vi "登陆界面.vi"(10 "引用":refnum<vi>) -> (1 "用户名":string, 2 "登陆状态":bool)   [LabVIEW 2014]
uses:
  Global.vi
panel:
  in  "退出":bool
  in  "登录":bool
  in  "密码":string
  in  "用户名":string
  # "（用户名为两位大写字母加数字组合）"
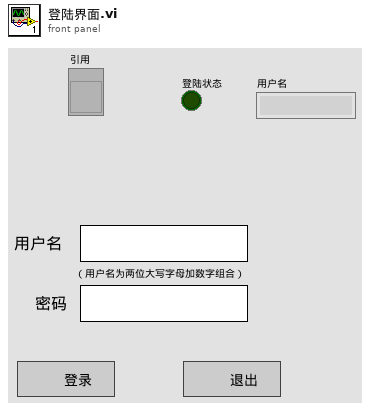
[diagram p1: front panel]
types:
  T1 = enum32{"Invalid", "Standard", "Closed", "Hidden", "Minimized", "Maximized"}
  T2 = enum8{"Enabled", "Disabled", "Disabled and Grayed Out"}
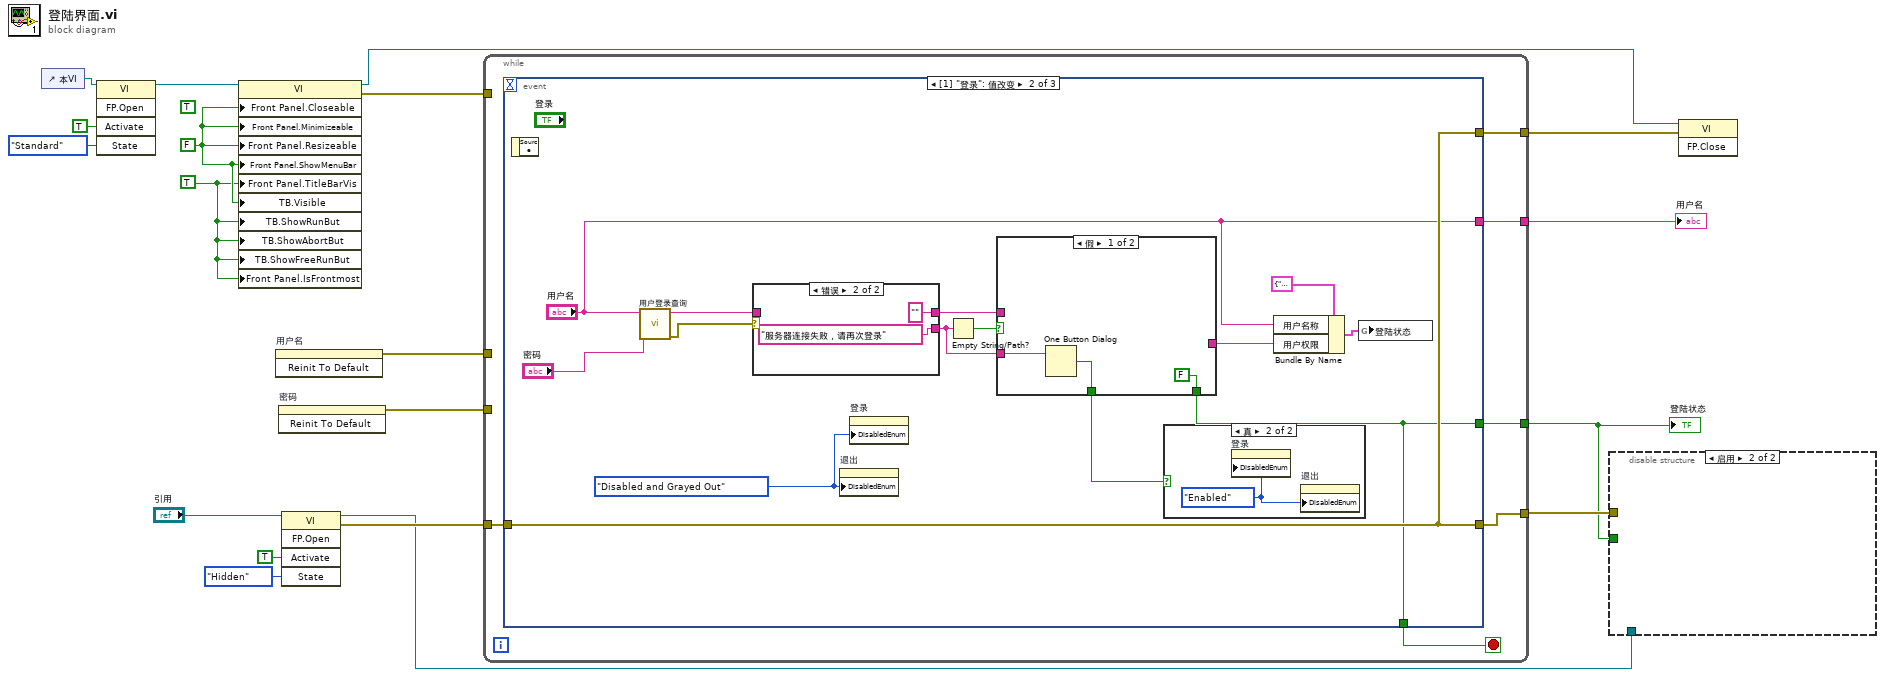
[diagram p0: block diagram]
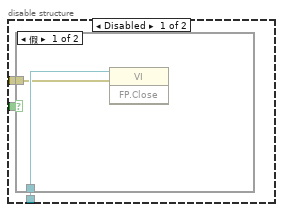
[diagram p2: hidden frame]
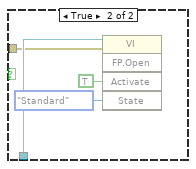
[diagram p3: hidden frame]
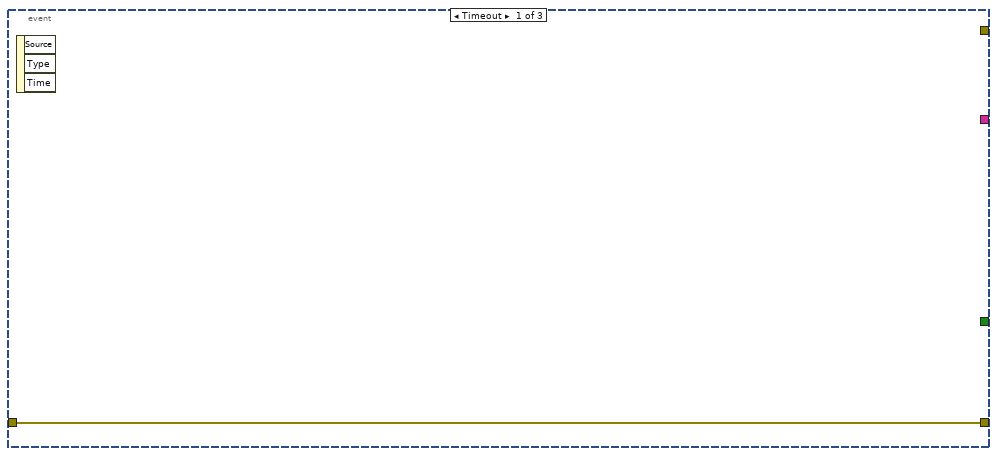
[diagram p4: hidden frame]
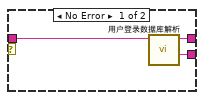
[diagram p6: hidden frame]
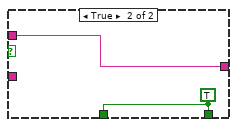
[diagram p7: hidden frame]
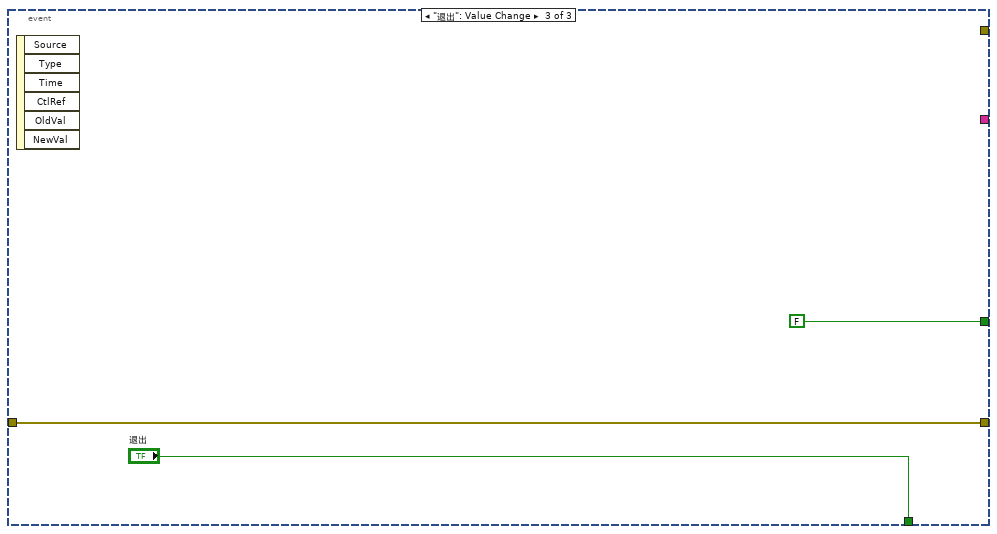
[diagram p8: hidden frame]
diagram:
  w11 = TRUE ("前面板窗口:可关闭")
  (unwired) TRUE ("前面板窗口:可关闭")
  w12 = FALSE ("Front Panel Window:Closeable")
  n1 = control-ref of="本VI"() -> (w10:refnum<vi>)
  n2 = invoke class="VI" method="FP.Open"(reference=w10, "Activate"=TRUE ("激活？"), "State"=T1."Standard" ("状态")) -> (reference out=w9:refnum<vi>)  [unwired: 2 in, 4 out]
  n3 = property class="VI"(reference=w9, "Front Panel.Closeable"=w12, "Front Panel.Minimizeable"=w12, "Front Panel.Resizeable"=w12, "Front Panel.ShowMenuBar"=w12, "Front Panel.TitleBarVis"=w11, "TB.Visible"=w12, "TB.ShowRunBut"=w11, "TB.ShowAbortBut"=w11, "TB.ShowFreeRunBut"=w11, "Front Panel.IsFrontmost"=w11) -> (reference out=w4:refnum<vi>, error out=w17:errorcluster)  [unwired: 1 in]
  n4 = invoke on="用户名" class="Str" method="Reinit To Default"() -> (error out=w19:errorcluster)  [unwired: 3 in, 2 out]
  n5 = invoke on="密码" class="Str" method="Reinit To Default"() -> (error out=w18:errorcluster)  [unwired: 3 in, 2 out]
  n6 = invoke class="VI" method="FP.Open"(reference="引用", "Activate"=TRUE ("激活？"), "State"=T1."Hidden" ("状态")) -> (reference out=w14:refnum<vi>, error out=w15:errorcluster)  [unwired: 2 in, 3 out]
  n7 = while {
    tunnel: [w24] -> w1
    tunnel: w19 -> [_]
    tunnel: w18 -> [_]
    tunnel: w17 -> [_]
    tunnel: w15 -> [w22]
    tunnel: [w23] -> w13
    tunnel: [w21] -> w3
    tunnel: [w20] -> w2
    stop <- w25 stop-if-true
    n8 = event shown="[1] \"登录\": 值改变" {
      selector: _ -> [_ _ _]
      dyn-events: _ -> [_ _ _]
      timeout: _ -> [_ _ _]
      tunnel: [_ w36 "退出"] -> w25
      tunnel: [_ w36 FALSE] -> w24
      tunnel: [w26 w38 w52] -> w23
      tunnel: w22 -> [w26 w38 w52]
      tunnel: [_ w38 _] -> w21
      tunnel: [_ "用户名" _] -> w20
      event Timeout {
        n9 = event-data() -> ()  [unwired: 1 in, 3 out]
      }
      event "登录": Value Change {
        w28 = T2."Disabled and Grayed Out" ("禁用")
        n10 = event-data() -> ()  [unwired: 1 in, 1 out]
        n11 = call "用户登录查询.vi"("密码"="密码", "用户名"="用户名") -> ("error out"=w30:errorcluster, "text"=w34:string)  [unwired: 8 in]
        n12 = case shown="错误" w30 {
          tunnel: w34 -> [w44 _]
          tunnel: [w43 "" ("权限")] -> w32
          tunnel: [w42 "服务器连接失败，请再次登录" ("异常信息")] -> w31
          frame No Error {
            n13 = call "用户登录数据库解析.vi"("text"=w44) -> ("异常信息"=w42:string, "权限"=w43:string)  [unwired: 9 in]
          }
          frame Error {
          }
        }
        n14 = property on="退出" class="Bool"("DisabledEnum"=w28) -> ()  [unwired: 2 in, 2 out]
        n15 = property on="登录" class="Bool"("DisabledEnum"=w28) -> ()  [unwired: 2 in, 2 out]
        n16 = Empty String/Path?(string/path=w31) -> (empty?=w33:bool)
        n17 = case shown="假" w33 {
          tunnel: [_ w51] -> w35
          tunnel: w32 -> [_ w51]
          tunnel: w31 -> [w49 _]
          tunnel: [FALSE w50] -> w36
          tunnel: [w47 w50] -> w29
          frame False {
            n18 = One Button Dialog(message=w49) -> (true=w47:bool)  [unwired: 1 in]
          }
          frame True {
            w50 = TRUE
          }
        }
        n19 = case shown="真" w29 {
          frame False {
          }
          frame True {
            w41 = T2."Enabled" ("禁用")
            n20 = property on="登录" class="Bool"("DisabledEnum"=w41) -> ()  [unwired: 2 in, 2 out]
            n21 = property on="退出" class="Bool"("DisabledEnum"=w41) -> ()  [unwired: 2 in, 2 out]
          }
        }
        n22 = Bundle By Name(cluster=cluster{"用户名称":string, "用户权限":string} {"用户名称"="", "用户权限"=""} ("登陆状态"), "用户名称"="用户名", "用户权限"=w35) -> (w39:cluster{"用户名称":string, "用户权限":string})
        n23 = global write "Global.vi" "登陆状态"(w39) -> ()
      }
      event "退出": Value Change {
        n24 = event-data() -> ()  [unwired: 1 in, 6 out]
      }
    }
  }
  "登陆状态" <- w1
  "用户名" <- w2
  n25 = disable-structure shown="启用" {
    disable-tunnel: w14 -> [w57 _]
    disable-tunnel: w13 -> [w56 _]
    disable-tunnel: w1 -> [w55 _]
    frame Disabled {
      n26 = case shown="假" w55 {
        tunnel: w57 -> [w59 w63]
        tunnel: w56 -> [w58 w62]
        frame False {
          n27 = invoke class="VI" method="FP.Close"(reference=w59, error in=w58) -> ()  [unwired: 1 in, 3 out]
        }
        frame True {
          n28 = invoke class="VI" method="FP.Open"(reference=w63, error in=w62, "Activate"=TRUE ("激活？"), "State"=T1."Standard" ("状态")) -> ()  [unwired: 1 in, 5 out]
        }
      }
    }
    frame Enabled {
    }
  }
  n29 = invoke class="VI" method="FP.Close"(reference=w4, error in=w3) -> ()  [unwired: 1 in, 3 out]
